vi "Write Precision.vi"(8 "error in (no error)":errorcluster, 10 "Precision":T1=enum."Nanoseconds", 11 "DataPoint in":refnum<class "DataPoint.lvclass">) -> (0 "error out":errorcluster, 3 "DataPoint out":refnum<class "DataPoint.lvclass">)   [LabVIEW 2018, in "InfluxDB Client.lvlib" / "DataPoint.lvclass"]
uses:
  DataPoint.lvclass
  Controls/Precision.ctl
  DataPoint.lvclass/DataPoint.ctl
  InfluxDB Client.lvlib
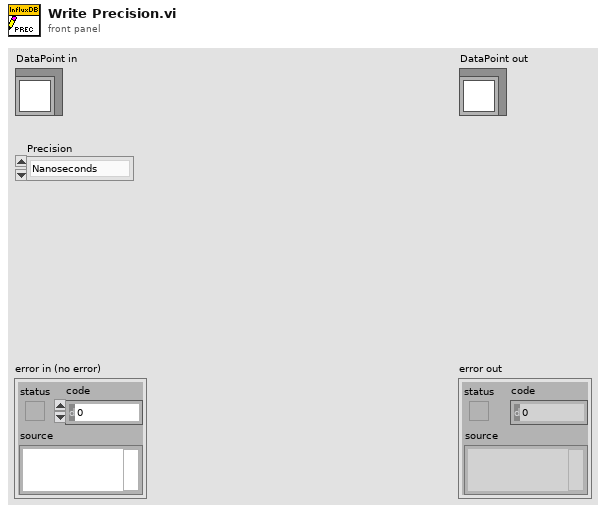
[diagram p1: front panel]
types:
  T1 = typedef "InfluxDB Client.lvlib/Precision.ctl" = enum16{"Seconds", "Milliseconds", "Nanoseconds"}
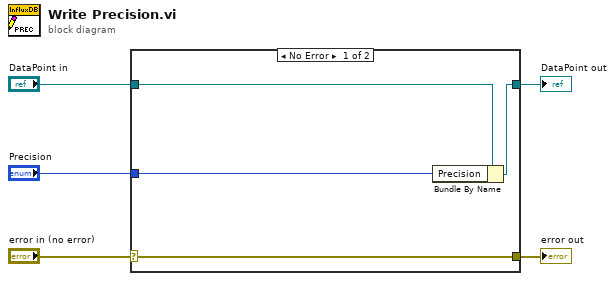
[diagram p0: block diagram]
diagram:
  n1 = case shown="No Error" "error in (no error)" {
    selector: "error in (no error)" -> [w9 w10]
    tunnel: [w9 w10] -> w4
    tunnel: [w7 w11] -> w2
    tunnel: "DataPoint in" -> [w8 w11]
    tunnel: "Precision" -> [w6 _]
    frame No Error {
      n2 = Bundle By Name(cluster=w8, "Precision"=w6) -> (w7:refnum<class "DataPoint.lvclass">)
    }
    frame Error {
    }
  }
  "error out" <- w4
  "DataPoint out" <- w2
